vi "Get Environment Activation String.vi"(8 "error in":errorcluster) -> (0 "error out":errorcluster, 3 "Conda Activation String":string)   [LabVIEW 2020, in "TALOS.lvlib" / "Kasli Wrapper 2.0.lvlib" / "Kasli Wrapper 2.0.lvclass"]
uses:
  Kasli Wrapper 2.0.lvclass
  Kasli/Kasli.lvclass
  Kasli Wrapper 2.0.lvlib
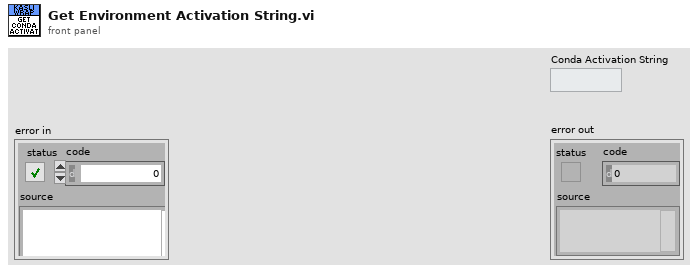
[diagram p1: front panel]
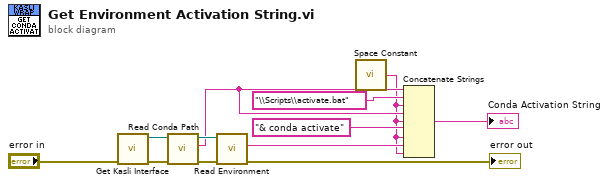
[diagram p0: block diagram]
diagram:
  n1 = call "Get Kasli Interface.vi"("error in"="error in") -> ("error out"=w12:errorcluster, "Kasli Interface"=w11:refnum<class "Kasli.lvclass">)  [unwired: 9 in]
  n2 = call-dynamic "Read Conda Path.vi"("error in (no error)"=w12, "Kasli in"=w11) -> ("error out"=w9:errorcluster, "Conda Path"=w6:string, "Kasli out"=w8:refnum<class "Kasli.lvclass">)  [unwired: 7 in]
  n3 = call-dynamic "Read Environment.vi"("error in (no error)"=w9, "Kasli in"=w8) -> ("error out"=→"error out":errorcluster, "Environment"=w4:string)  [unwired: 7 in, 1 out]
  n4 = call <vilib>:"Space Constant.vi"() -> ("String"=w3:string)
  n5 = Concatenate Strings(w6, "\\Scripts\\activate.bat" ("string"), w3, w6, w3, "& conda activate" ("standard input"), w3, w4, w3) -> (→"Conda Activation String":string)
